vi "Parse Status Channels.vi"(5 "FIFO Idx Qs":T2, 8 "error in":errorcluster, 11 "Device Reference in":T1 format="%.0x") -> (0 "error out":errorcluster, 2 "Status Config":T3 {"HWOut Dur Ref" format="%.0x"; "HWIn Dur Ref" format="%.0x"; "Error Data Ref" format="%.0x"}, 3 "Device Ref out":T1 format="%.0x")   [LabVIEW 2016, in "Ballard Arinc-429 Engine.lvlib"]
uses:
  Ballard Arinc-429 Engine.lvlib
  RT Controls/Status Channels Config.ctl
  <vilib>/NI Veristand/Custom Device API/Data Reference.ctl
  RT Controls/FIFO Idx Qs.ctl
  <vilib>/NI Veristand/Custom Device API/Custom Device Item Ref.ctl
  <vilib>/NI Veristand/Custom Device API/Data Access Type.ctl
  RT Controls/Data Ref FGV Command.ctl
  <vilib>/NI Veristand/Custom Device Tools/Custom Device Utility Library/NI VeriStand - Search for Item by Name.vi
  Shared/Controls and Global/Global.vi
  <vilib>/NI Veristand/Custom Device Tools/Custom Device Utility Library/Custom Device Utility Library.lvlib
  Shared/Ballard Arinc-429 Shared.lvlib
  <vilib>/NI Veristand/Custom Device API/Custom Device API.lvlib
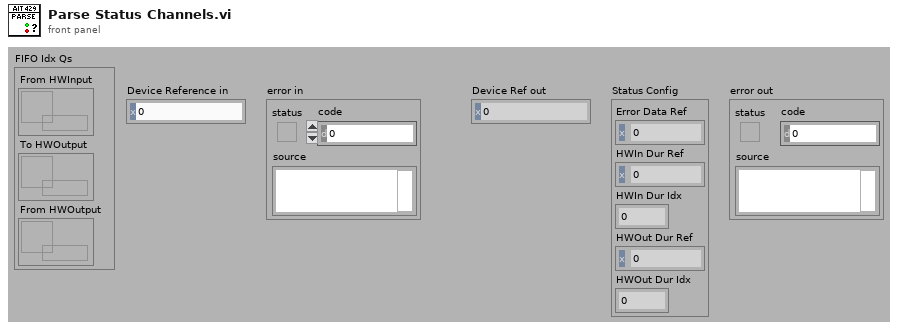
[diagram p1: front panel]
types:
  T1 = typedef "Custom Device API.lvlib/Custom Device Item Ref.ctl" = u64
  T2 = typedef "Ballard Arinc-429 Engine.lvlib/FIFO Idx Qs.ctl" = cluster{"From HWInput":refnum<queue>, "To HWOutput":refnum<queue>, "From HWOutput":refnum<queue>}
  T3 = typedef "Ballard Arinc-429 Engine.lvlib/Status Channels Config.ctl" = cluster{"Error Data Ref":T4, "HWIn Dur Ref":T4, "HWIn Dur Idx":i32, "HWOut Dur Ref":T4, "HWOut Dur Idx":i32}
  T4 = typedef "Custom Device API.lvlib/Data Reference.ctl" = i32
  T5 = typedef "Ballard Arinc-429 Engine.lvlib/Data Ref FGV Command.ctl" = enum16{"Intialize", "Get", "Update"}
  T6 = typedef "Custom Device API.lvlib/Data Access Type.ctl" = enum16{"Read", "Write"}
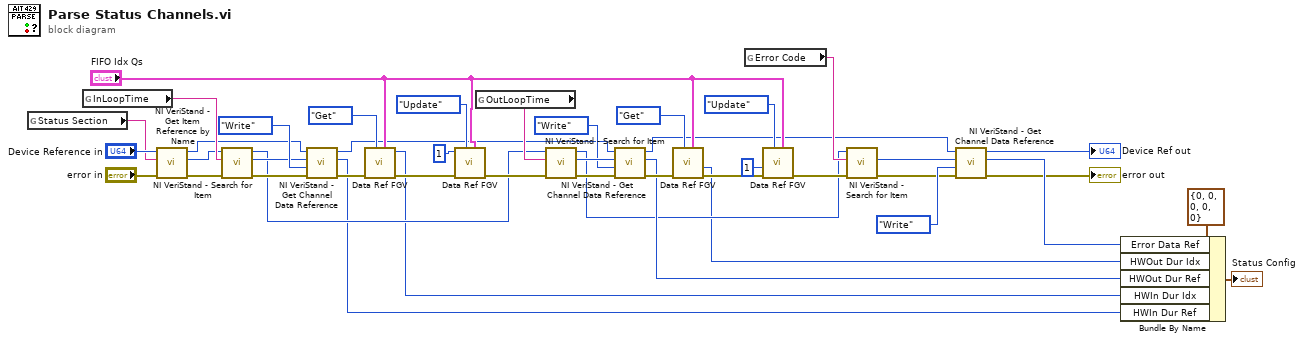
[diagram p0: block diagram]
diagram:
  n1 = global read "Global.vi" "Status Section"() -> (w34:string)
  n2 = global read "Global.vi" "InLoopTime"() -> (w32:string)
  n3 = call <vilib>:"NI VeriStand - Get Item Reference by Name.vi"("error in (no error)"="error in", "Item Name"=w34, "Parent Ref in"="Device Reference in") -> ("error out"=w15:errorcluster, "Item Ref"=w16:T1, "Parent Ref out"=w14:T1)  [unwired: 5 in, 1 out]
  n4 = call-poly <vilib>:"NI VeriStand - Search for Item.vi"("error in"=w15, "Item Name"=w32, "Section Ref in"=w16) -> ("error out"=w30:errorcluster, "Item Ref"=w29:T1, "Section Ref out"=w10:T1)  [unwired: 5 in, 1 out]
  n5 = call <vilib>:"NI VeriStand - Get Channel Data Reference.vi"("error in (no error)"=w30, "Access"=Data_Access_Type."Write", "Channel Ref in"=w29, "Device Ref in"=w14) -> ("error out"=w28:errorcluster, "Channel Data Reference"=w5:T4, "Device Ref out"=w8:T1)  [unwired: 5 in]
  n6 = call "Data Ref FGV.vi"("FIFO Idx Qs"="FIFO Idx Qs", "Command"=Data_Ref_FGV_Command."Get", "error in (no error)"=w28) -> ("error out"=w26:errorcluster, "From HWInput FIFO Index / Length"=w6:i32)  [unwired: 5 in, 2 out]
  n7 = call "Data Ref FGV.vi"("FIFO Idx Qs"="FIFO Idx Qs", "Command"=Data_Ref_FGV_Command."Update", "error in (no error)"=w26, "From HWInput Length"=1 ("HWInput Length")) -> ("error out"=w13:errorcluster)  [unwired: 4 in, 3 out]
  n8 = global read "Global.vi" "OutLoopTime"() -> (w17:string)
  n9 = call-poly <vilib>:"NI VeriStand - Search for Item.vi"("error in"=w13, "Item Name"=w17, "Section Ref in"=w10) -> ("error out"=w19:errorcluster, "Item Ref"=w20:T1, "Section Ref out"=w3:T1)  [unwired: 5 in, 1 out]
  n10 = call <vilib>:"NI VeriStand - Get Channel Data Reference.vi"("error in (no error)"=w19, "Access"=Data_Access_Type."Write", "Channel Ref in"=w20, "Device Ref in"=w8) -> ("error out"=w21:errorcluster, "Channel Data Reference"=w7:T4, "Device Ref out"=w4:T1)  [unwired: 5 in]
  n11 = call "Data Ref FGV.vi"("FIFO Idx Qs"="FIFO Idx Qs", "Command"=Data_Ref_FGV_Command."Get", "error in (no error)"=w21) -> ("error out"=w23:errorcluster, "From HWOutput FIFO Index / Length"=w2:i32)  [unwired: 5 in, 2 out]
  n12 = global read "Global.vi" "Error Code"() -> (w33:string)
  n13 = call "Data Ref FGV.vi"("FIFO Idx Qs"="FIFO Idx Qs", "Command"=Data_Ref_FGV_Command."Update", "error in (no error)"=w23, "From HWOutput Length"=1 ("HWInput Length")) -> ("error out"=w12:errorcluster)  [unwired: 4 in, 3 out]
  n14 = call-poly <vilib>:"NI VeriStand - Search for Item.vi"("error in"=w12, "Item Name"=w33, "Section Ref in"=w3) -> ("error out"=w37:errorcluster, "Item Ref"=w40:T1)  [unwired: 5 in, 2 out]
  n15 = call <vilib>:"NI VeriStand - Get Channel Data Reference.vi"("error in (no error)"=w37, "Access"=Data_Access_Type."Write", "Channel Ref in"=w40, "Device Ref in"=w4) -> ("error out"=→"error out":errorcluster, "Channel Data Reference"=w43:T4, "Device Ref out"=→"Device Ref out":T1)  [unwired: 5 in]
  n16 = Bundle By Name(cluster=T3 {"Error Data Ref"=0, "HWIn Dur Ref"=0, "HWIn Dur Idx"=0, "HWOut Dur Ref"=0, "HWOut Dur Idx"=0} ("Stat Chn Cfg"), "Error Data Ref"=w43, "HWOut Dur Idx"=w2, "HWOut Dur Ref"=w7, "HWIn Dur Idx"=w6, "HWIn Dur Ref"=w5) -> (→"Status Config":T3)
